vi "AccelMonitor.vi"() -> ()   [LabVIEW 2013]
panel:
  out "Waveform Chart":i32[](graph)
  in  "?":bool
  out "Acceleration out of Range":bool
  in  "Min Acceleration":i32=15
  in  "Max Acceleration":i32=30
  out "Ch8":i32
  out "Ch7":i32
  out "Ch6":i32
  out "Ch5":i32
  out "Ch4":i32
  out "Ch3":i32
  out "Ch2":i32
  out "Ch1":i32
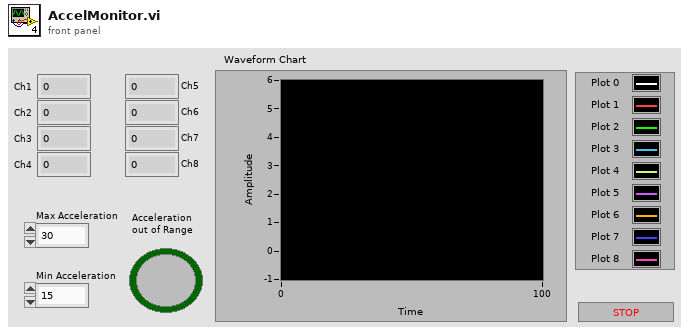
[diagram p1: front panel]
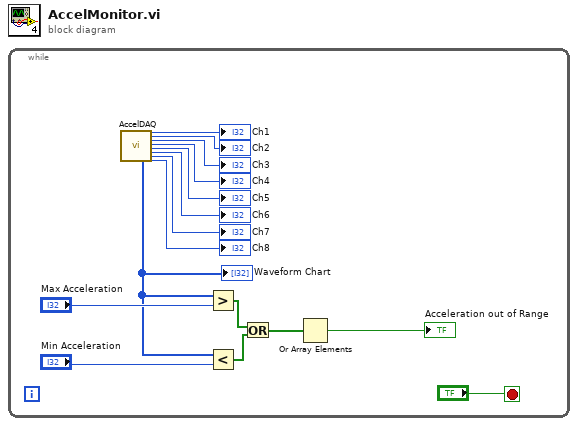
[diagram p0: block diagram]
diagram:
  n1 = while {
    stop <- "?" stop-if-true
    n2 = call "AccelDAQ.vi"() -> ("AccelArray"=w1:i32[], "element_1"=→"Ch1":i32, "element_2"=→"Ch2":i32, "element_3"=→"Ch3":i32, "element_4"=→"Ch4":i32, "element_5"=→"Ch5":i32, "element_6"=→"Ch6":i32, "element_7"=→"Ch7":i32, "element_8"=→"Ch8":i32)  [unwired: 19 in]
    "Waveform Chart" <- w1
    n3 = Greater?(x=w1, y="Max Acceleration") -> (0:w6:bool[])
    n4 = Less?(x=w1, y="Min Acceleration") -> (x < y?=w5:bool[])
    n5 = Or(x=w6, y=w5) -> (x .or. y?=w4:bool[])
    n6 = Or Array Elements(Boolean array=w4) -> (logical OR=→"Acceleration out of Range":bool)
  }
